vi "DPT Gas Flow Readings.vi"(0 "Com Flow Computer":refnum<visa-resource-name>, 1 "task/channels in":refnum<k21>="PortRead", 5 "Use SL9200 Gas Readings?":bool, 7 "Use Dry Gas Meter?":bool=TRUE, 9 "Initialize?":bool=TRUE, 11 "Error In":errorcluster, 12 "Encoder":T1={"ft3 Per Rotation"=0.1, "Ticks Per Rotation"=400.0, "Data Sample Period(mS)"=10, "Number of Samples"=50} {"ft3 Per Rotation" format="%_3g"}) -> (4 "Labels":string[](array[string]), 6 "Values":string[](array[string]), 15 "error out":errorcluster)   [LabVIEW 2016]
uses:
  Drivers/SL9200/Type Definitions/SL9200 Registers.ctl
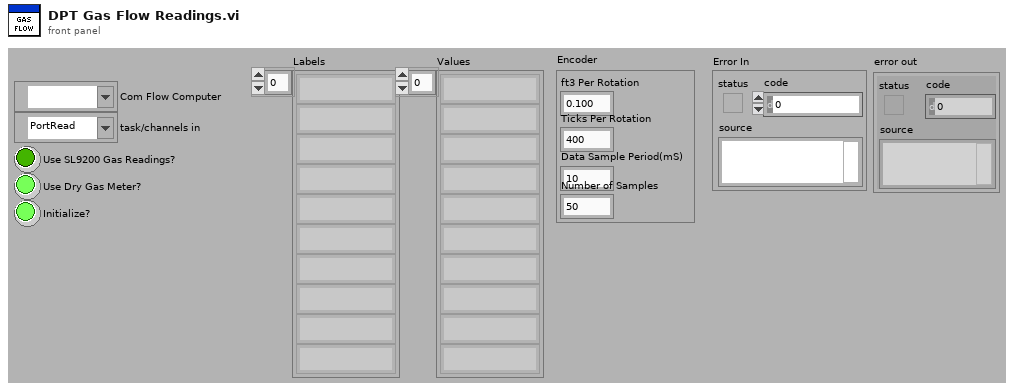
[diagram p1: front panel]
types:
  T1 = cluster{"ft3 Per Rotation":dbl, "Ticks Per Rotation":dbl, "Data Sample Period(mS)":u32, "Number of Samples":i32}
  T2 = typedef "SL9200 Registers.ctl" = u8
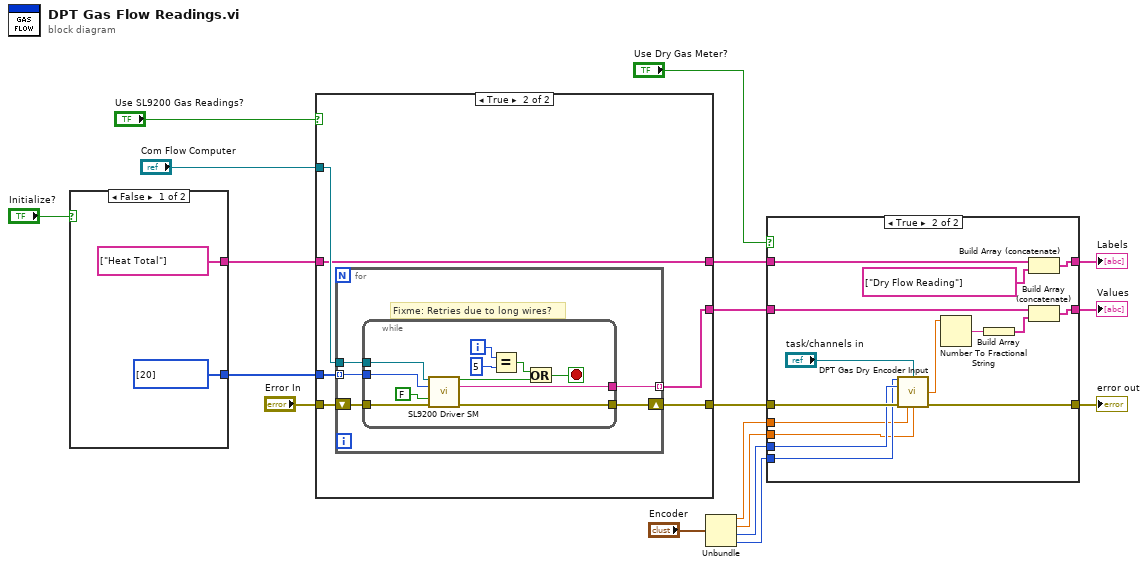
[diagram p0: block diagram]
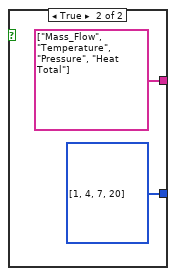
[diagram p3: hidden frame]
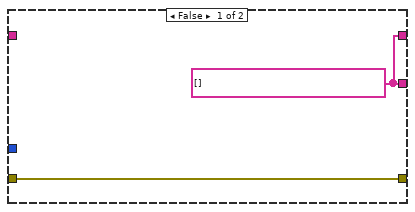
[diagram p4: hidden frame]
diagram:
  n1 = case shown="False" "Initialize?" {
    tunnel: [w20 w22] -> w17
    tunnel: [string[] ["Heat Total"] ("array") string[] ["Mass_Flow", "Temperature", "Pressure", "Heat Total"] ("array")] -> w18
    frame False {
      w20 = T2[] [20] items=["Heat_Flow", "Mass_Flow", "Corrected_Volume_Flow", "Volume_Flow", "Temperature", "Temperature2", "Delta_Temperature", "Pressure", "Diff_Pressure", "Density", "Spec_Enthalpy", "Date", "Time", "Level", "Peak_Demand", "Demand_Last_Hour", "Peak_Demand_Time", "Peak_Demand_Date", "Viscosity", "Reynolds_Number", "Heat_Total", "Grand_Heat_Total", "Mass_Total", "Grand_Mass", "Corrected_Volume_Total", "Grand_Corrected_Volume", "Volume_Total", "Grand_Volume", "Totalizer_Reset", "Alarm_Reset", "Barometric", "Fluid_Type", "Reference_Density", "Therm_Expansion_Coef", "Combustion_Heat", "Specific_Heat", "Flow_Z_Factor", "Ref_Z_Factor", "Isentropic_Exponent", "Viscosity_A", "Viscosity_B", "Reference_Temperature", "Calibration_Density", "Base_Density_H2O_4C", "Per_Mole_N2", "Per_Mole_CO2", "Tag_Number", "Software_Version", "Hardware_Version", "Order_Code", "Serial_Number", "Sensor_Serial_Num"]
    }
    frame True {
      w22 = T2[] [1, 4, 7, 20] items=["Heat_Flow", "Mass_Flow", "Corrected_Volume_Flow", "Volume_Flow", "Temperature", "Temperature2", "Delta_Temperature", "Pressure", "Diff_Pressure", "Density", "Spec_Enthalpy", "Date", "Time", "Level", "Peak_Demand", "Demand_Last_Hour", "Peak_Demand_Time", "Peak_Demand_Date", "Viscosity", "Reynolds_Number", "Heat_Total", "Grand_Heat_Total", "Mass_Total", "Grand_Mass", "Corrected_Volume_Total", "Grand_Corrected_Volume", "Volume_Total", "Grand_Volume", "Totalizer_Reset", "Alarm_Reset", "Barometric", "Fluid_Type", "Reference_Density", "Therm_Expansion_Coef", "Combustion_Heat", "Specific_Heat", "Flow_Z_Factor", "Ref_Z_Factor", "Isentropic_Exponent", "Viscosity_A", "Viscosity_B", "Reference_Temperature", "Calibration_Density", "Base_Density_H2O_4C", "Per_Mole_N2", "Per_Mole_CO2", "Tag_Number", "Software_Version", "Hardware_Version", "Order_Code", "Serial_Number", "Sensor_Serial_Num"]
    }
  }
  n2 = case shown="True" "Use SL9200 Gas Readings?" {
    tunnel: w17 -> [_ w30]
    tunnel: "Error In" -> [w24 w29]
    tunnel: "Com Flow Computer" -> [_ w28]
    tunnel: [w24 w27] -> w1
    tunnel: [w23 w26] -> w2
    tunnel: [w23 w25] -> w3
    tunnel: w18 -> [_ w25]
    frame False {
      w23 = string[] [] ("array")
    }
    frame True {
      n3 = for {
        tunnel: w28 -> [w35]
        tunnel: [w34] -> w26 mode=indexing
        tunnel: w30 -> [w33] mode=indexing
        shift-right: [w31] -> w27
        shift-left: w29 -> [w32]
        # "Fixme: Retries due to long wires?"
        n4 = while {
          tunnel: w35 -> [w46]
          tunnel: [w45] -> w34
          tunnel: w33 -> [w44]
          tunnel: w32 -> [w43]
          tunnel: [w42] -> w31
          i -> [w39]
          stop <- w36 stop-if-true
          n5 = call "SL9200 Driver SM.vi"("ComPort"=w46, "Register"=w44, "InitSerial?"=FALSE, "Error In"=w43) -> ("CMD OK"=w40:bool, "Response"=w45:string, "Error Out"=w42:errorcluster)  [unwired: 9 in]
          n6 = Equal?(x=w39, y=5) -> (x = y?=w37:bool)
          n7 = Or(x=w37, y=w40) -> (x .or. y?=w36:bool)
        }
      }
    }
  }
  n8 = Unbundle("Encoder") -> ("ft3 Per Rotation"=w15:dbl, "Ticks Per Rotation"=w16:dbl, "Data Sample Period(mS)"=w13:u32, "Number of Samples"=w14:i32)
  n9 = case shown="True" "Use Dry Gas Meter?" {
    tunnel: w1 -> [w49 w64]
    tunnel: w3 -> [w47 w63]
    tunnel: [w47 w60] -> w9
    tunnel: w2 -> [w48 w59]
    tunnel: [w48 w58] -> w11
    tunnel: [w49 w55] -> w10
    tunnel: w13 -> [_ w53]
    tunnel: w14 -> [_ w52]
    tunnel: w15 -> [_ w51]
    tunnel: w16 -> [_ w50]
    frame False {
    }
    frame True {
      n10 = call "DPT Gas Dry Encoder Input.vi"("Number of Samples"=w52, "task/channels in"="task/channels in", "Data Sample Period(mS)"=w53, "error in (no error)"=w64, "ft3 Per Rotation"=w51, "Ticks Per Rotation"=w50) -> ("ft3 per Hour"=w61:dbl, "error out"=w55:errorcluster)  [unwired: 6 in, 2 out]
      n11 = Number To Fractional String(number=w61) -> (F-format string=w56:string)  [unwired: 3 in]
      n12 = Build Array(w56) -> (w57:string[])
      n13 = Build Array (concatenate)(w63, string[] ["Dry Flow Reading"] ("array")) -> (w60:string[])
      n14 = Build Array (concatenate)(w59, w57) -> (w58:string[])
    }
  }
  "error out" <- w10
  "Labels" <- w9
  "Values" <- w11
